vi "sub vi - Move Piezo Stage.vi"(6 "stop":bool, 8 "Frequency":dbl=0.5 min=0.0, 9 "Desired Position (um)":dbl min=0.0 max=12.0 format="%0.2f", 10 "Axis":u16(ring) items=["X", "Y", "Z"], 11 "All Axis":bool) -> (1 "Z Position":dbl, 2 "Y Position":dbl, 3 "X Position":dbl)   [LabVIEW 2010]
uses:
  <vilib>/DAQmx/write.llb/DAQmx Write (Analog DBL 1Chan 1Samp).vi
  <vilib>/DAQmx/create/channels.llb/DAQmx Create Channel (AO-Voltage-Basic).vi
  <vilib>/daqmx/miscellaneous.llb/DAQmx Fill In Error Info.vi
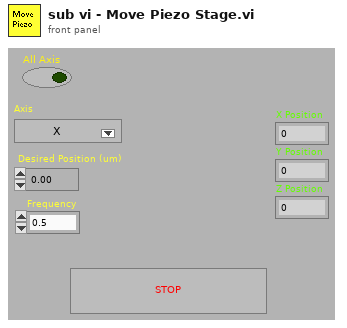
[diagram p1: front panel]
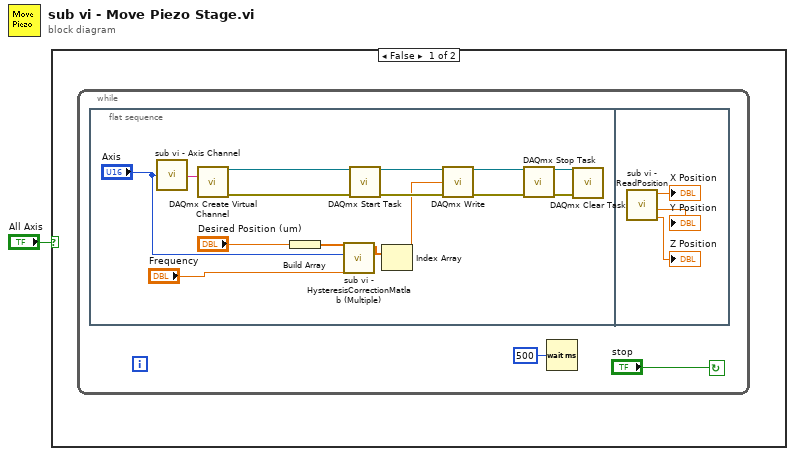
[diagram p0: block diagram]
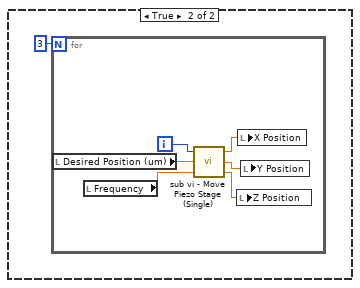
[diagram p2: hidden frame]
diagram:
  n1 = case shown="False" "All Axis" {
    frame False {
      n2 = while {
        stop <- "stop" continue-if-true
        n3 = flat-sequence {
          frame #0 {
            n4 = call "sub vi - Axis Channel.vi"("Axis"="Axis") -> ("physical channels"=w10:tag)
            n5 = call-poly <vilib>:"DAQmx Create Virtual Channel.vi"("physical channels"=w10) -> ("task out"=w18:refnum<k21>, "error out"=w17:errorcluster)  [unwired: 8 in, 5 out]
            n6 = Build Array("Desired Position (um)") -> (w4:dbl[])
            n7 = call "sub vi - HysteresisCorrectionMatlab (Multiple).vi"("frequency"="Frequency", "Axis"="Axis", "desired positions"=w4) -> ("correctV"=w6:dbl[])  [unwired: 8 out]
            n8 = call <vilib>:"DAQmx Start Task.vi"("task/channels in"=w18, "error in"=w17) -> ("task out"=w14:refnum<k21>, "error out"=w11:errorcluster)  [unwired: 12 out]
            n9 = Index Array(array=w6) -> (element=w5:dbl)  [unwired: 1 in]
            n10 = call-poly <vilib>:"DAQmx Write.vi"("task/channels in"=w14, "data"=w5, "error in"=w11) -> ("task out"=w13:refnum<k21>, "error out"=w12:errorcluster)  [unwired: 1 in, 10 out]
            n11 = call <vilib>:"DAQmx Stop Task.vi"("task/channels in"=w13, "error in"=w12) -> ("task out"=w16:refnum<k21>, "error out"=w15:errorcluster)  [unwired: 12 out]
            n12 = call <vilib>:"DAQmx Clear Task.vi"("task in"=w16, "error in"=w15) -> ()  [unwired: 14 out]
          }
          frame #1 {
            n13 = call "sub vi - ReadPosition.vi"() -> ("Z Position"=→"Z Position":dbl, "Y Position"=→"Y Position":dbl, "X Position"=→"X Position":dbl)  [unwired: 9 out]
          }
        }
        n14 = Wait (ms)(milliseconds to wait=u32 500) -> ()  [unwired: 1 out]
      }
    }
    frame True {
      n15 = for {
        N: 3 -> [_]
        i -> [w28]
        n16 = local read "Desired Position (um)"() -> (w25:dbl)
        n17 = local read "Frequency"() -> (w26:dbl)
        n18 = call "sub vi - Move Piezo Stage (Single).vi"("frequency"=w26, "Desired Position (um)"=w25, "Axis"=w28) -> ("Z Position"=w23:dbl, "Y Position"=w24:dbl, "X Position"=w27:dbl)
        n19 = local write "Z Position"(w23) -> ()
        n20 = local write "X Position"(w27) -> ()
        n21 = local write "Y Position"(w24) -> ()
      }
    }
  }
